vi "Actor Core.vi"(8 "error in":errorcluster, 11 "Pic Json Generator in":refnum<class "Pic Json Generator.lvclass">) -> (0 "error out":errorcluster, 3 "Actor out":refnum<class "Actor.lvclass">)   [LabVIEW 2018, in "Pic Json Generator.lvlib" / "Pic Json Generator.lvclass"]
doc: "The user interface for this panel.\n\n----\nPlease see the following web address for additional documentation and tutorial information:\nhttp://www.mooregoodideas.com/mgi-panel-manager/\n\nAuthor: Derek Trepanier\n\nCopyright (c) 2018, Moore Good Ideas, Inc.\n\nAll rights reserved.\n\nRedistribution and use in source and binary forms, with or without modification, are permitted provided that the following conditions are met:\n\n * Redistributions of source code must retain the above copyright notice, this list of conditions and the following disclaimer.\n * Redistributions in binary form must reproduce the above copyright notice, this list of conditions and the following disclaimer in the documentation and/or other materials provided with the distribution.\n * Neither the name of Moore Good Ideas, Inc. nor the names of its contributors may be used to endorse or promote products derived from this software without specific prior written permission.\n\nTHIS SOFTWARE IS PROVIDED BY THE COPYRIGHT HOLDERS AND CONTRIBUTORS \"AS IS\" AND ANY EXPRESS OR IMPLIED WARRANTIES, INCLUDING, BUT NOT LIMITED TO, THE IMPLIED WARRANTIES OF MERCHANTABILITY AND FITNESS FOR A PARTICULAR PURPOSE ARE DISCLAIMED. IN NO EVENT SHALL THE COPYRIGHT OWNER OR CONTRIBUTORS BE LIABLE FOR ANY DIRECT, INDIRECT, INCIDENTAL, SPECIAL, EXEMPLARY, OR CONSEQUENTIAL DAMAGES (INCLUDING, BUT NOT LIMITED TO, PROCUREMENT OF SUBSTITUTE GOODS OR SERVICES; LOSS OF USE, DATA, OR PROFITS; OR BUSINESS INTERRUPTION) HOWEVER CAUSED AND ON ANY THEORY OF LIABILITY, WHETHER IN CONTRACT, STRICT LIABILITY, OR TORT (INCLUDING NEGLIGENCE OR OTHERWISE) ARISING IN ANY WAY OUT OF THE USE OF THIS SOFTWARE, EVEN IF ADVISED OF THE POSSIBILITY OF SUCH DAMAGE."
uses:
  Pic Json Generator.lvclass
  C:/Program Files (x86)/National Instruments/LabVIEW 2018/vi.lib/MGI/Panel Manager/Panel Actor/Panel Actor/Panel Actor.lvclass
  C:/Program Files (x86)/National Instruments/LabVIEW 2018/vi.lib/ActorFramework/Actor/Actor.lvclass
  <vilib>/ActorFramework/Actor/Actor.lvclass
  Pic Json Generator.lvclass/Pic Json Generator.ctl
  <vilib>/ActorFramework/Actor/Actor.lvclass/Actor.ctl
  <vilib>/ActorFramework/Message Enqueuer/Message Enqueuer.lvclass/Message Enqueuer.ctl
  <vilib>/ActorFramework/Message Enqueuer/Init from Existing Queue.vi
  <vilib>/ActorFramework/Message Enqueuer/Enqueue.vi
  <vilib>/ActorFramework/Stop Msg/Stop Msg.lvclass
  C:/Program Files (x86)/National Instruments/LabVIEW 2018/vi.lib/ActorFramework/Message/Message.lvclass
  <vilib>/ActorFramework/Message Priority Queue/Priority Enqueue.vi
  <vilib>/ActorFramework/Message Enqueuer/Message Enqueuer.lvclass
  <vilib>/MGI/Panel Manager/Panel Actor/Panel Actor/Panel Actor.lvclass
panel:
  out "Frame Height":u32
  out "Frame Width":u32
  out "End Frame Num":u32
  in  "Generate":bool
  in  "Start Frame Num":u32
  in  "Num of Row":u32
  in  "Num of Column":u32
  in  "Pic File Path":path
  in  "Data File Path":path
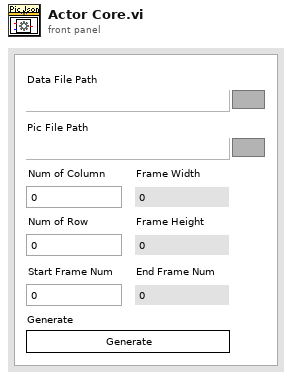
[diagram p1: front panel]
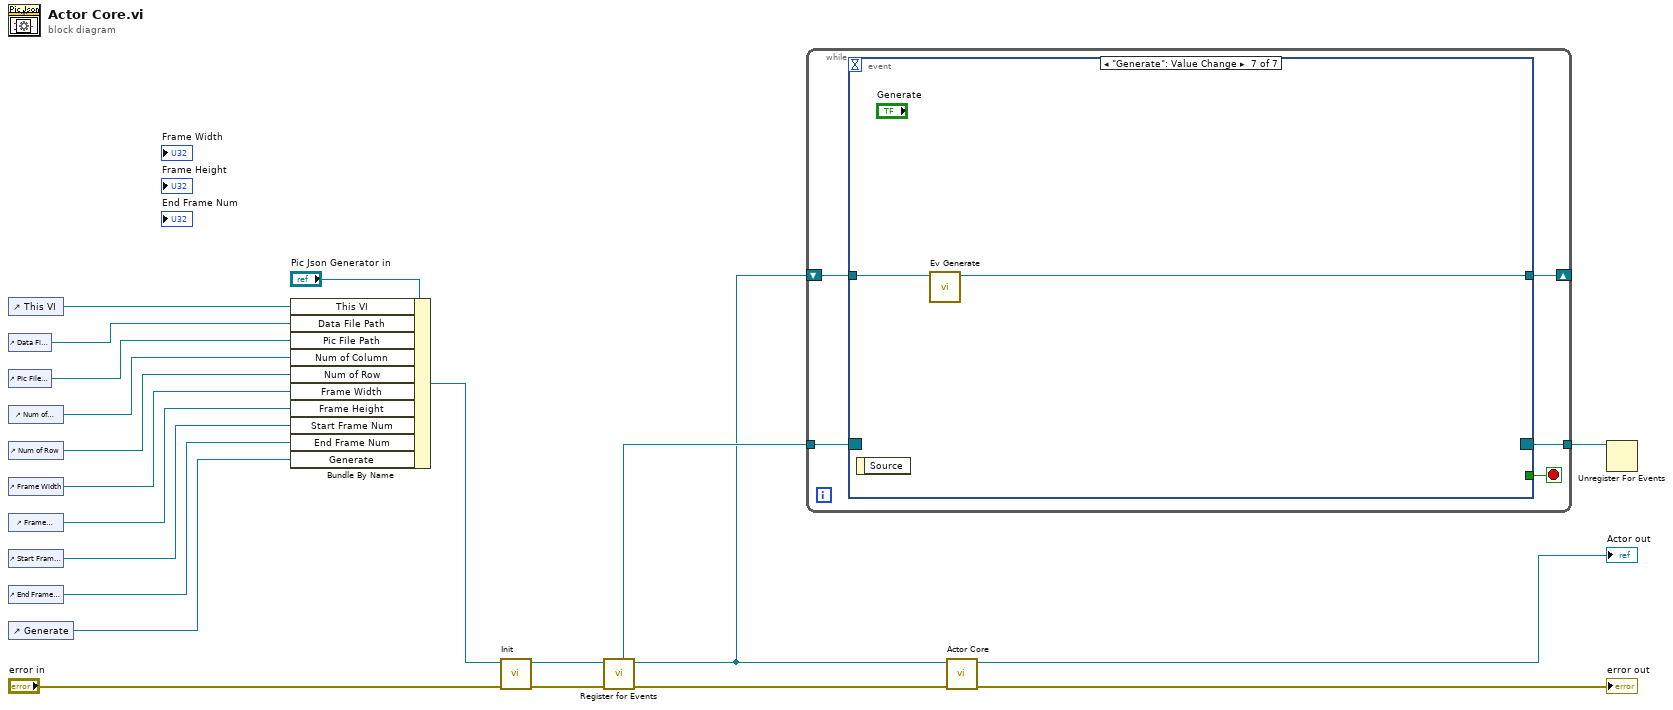
[diagram p0: block diagram]
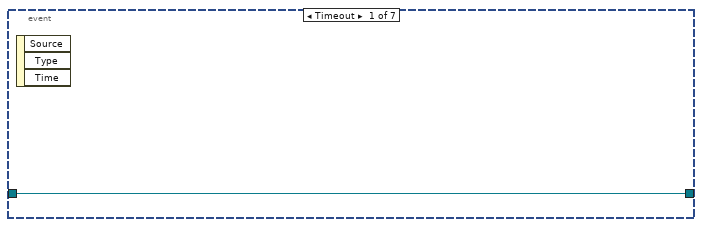
[diagram p2: hidden frame]
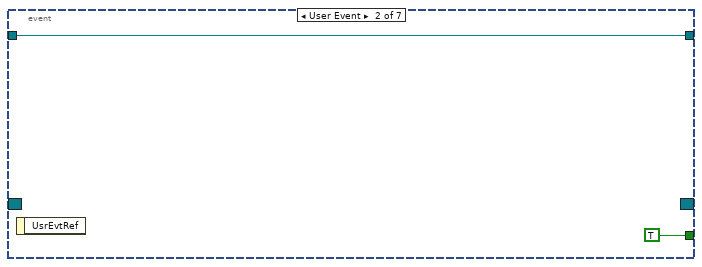
[diagram p3: hidden frame]
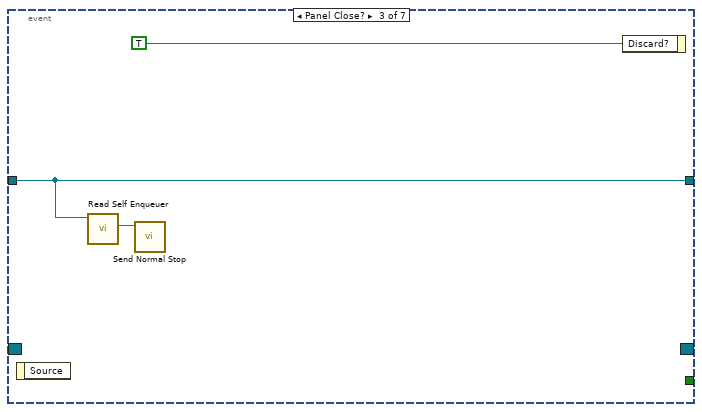
[diagram p4: hidden frame]
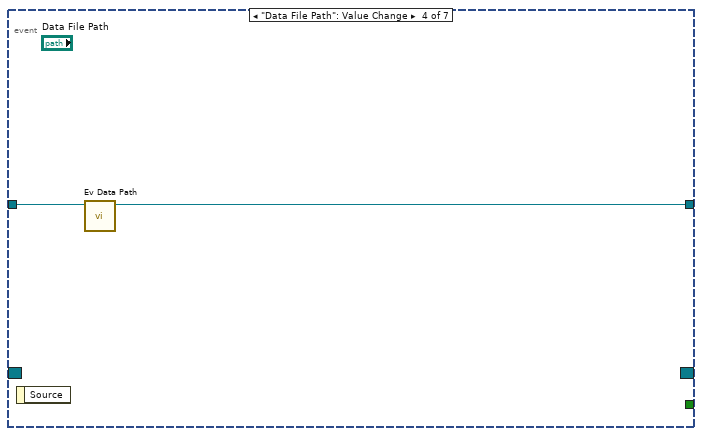
[diagram p5: hidden frame]
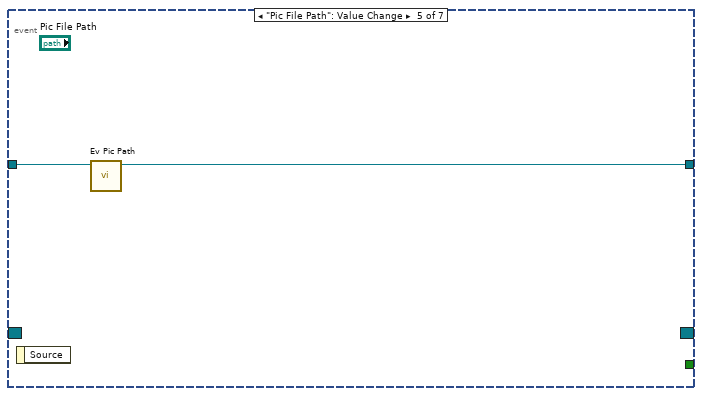
[diagram p6: hidden frame]
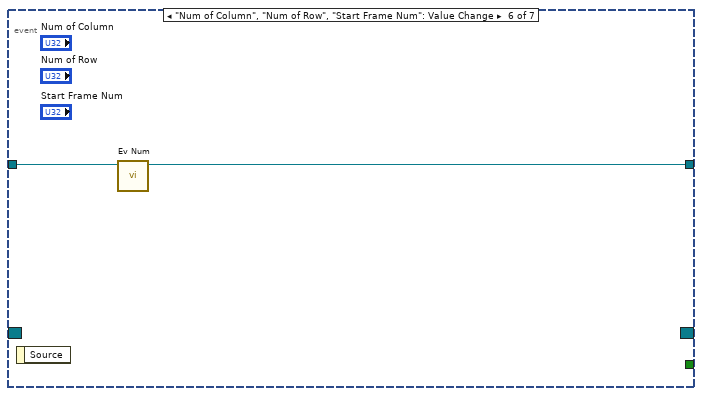
[diagram p7: hidden frame]
diagram:
  n1 = control-ref of="This VI"() -> (w1:refnum<vi>)
  n2 = control-ref of="Data File Path"() -> (w11:refnum<vi>)
  n3 = control-ref of="Pic File Path"() -> (w10:refnum<vi>)
  n4 = control-ref of="Num of Column"() -> (w7:refnum<vi>)
  n5 = control-ref of="Num of Row"() -> (w6:refnum<vi>)
  n6 = control-ref of="Frame Width"() -> (w5:refnum<vi>)
  n7 = control-ref of="Frame Height"() -> (w4:refnum<vi>)
  n8 = control-ref of="Start Frame Num"() -> (w3:refnum<vi>)
  n9 = control-ref of="End Frame Num"() -> (w2:refnum<vi>)
  n10 = control-ref of="Generate"() -> (w9:refnum<vi>)
  n11 = Bundle By Name(cluster="Pic Json Generator in", "This VI"=w1, "Data File Path"=w11, "Pic File Path"=w10, "Num of Column"=w7, "Num of Row"=w6, "Frame Width"=w5, "Frame Height"=w4, "Start Frame Num"=w3, "End Frame Num"=w2, "Generate"=w9) -> (w8:refnum<class "Pic Json Generator.lvclass">)
  n12 = call "Init.vi"("error in (no error)"="error in", "Pic Json Generator in"=w8) -> ("error out"=w17:errorcluster, "Pic Json Generator out"=w18:refnum<class "Pic Json Generator.lvclass">)  [unwired: 8 in]
  n13 = call <vilib>:"Register for Events.vi"("Error In"=w17, "Panel Actor in"=w18) -> ("Error Out"=w16:errorcluster, "Panel Actor out"=w13:refnum<class "Pic Json Generator.lvclass">, "Pnl Actor"=w14:refnum<event-registration>)  [unwired: 6 in, 1 out]
  n14 = while {
    tunnel: w14 -> [w26]
    tunnel: [w24] -> w15
    shift-right: [w22] -> _
    shift-left: w13 -> [w23]
    stop <- w25 stop-if-true
    n15 = event shown="[6] \"Generate\": Value Change" {
      selector: w26 -> [_ _ _ _ _ _ _]
      dyn-events: [_ _ _ _ _ _ _] -> w24
      timeout: _ -> [_ _ _ _ _ _ _]
      tunnel: [_ TRUE _ _ _ _ _] -> w25
      tunnel: w23 -> [w27 w28 w30 w34 w36 w38 w40]
      tunnel: [w27 w28 w30 w33 w35 w37 w39] -> w22
      event Timeout {
        n16 = event-data() -> ()  [unwired: 1 in, 3 out]
      }
      event User Event {
        n17 = event-data() -> ()  [unwired: 1 in, 1 out]
      }
      event Panel Close? {
        n18 = event-data() -> ()  [unwired: 1 in, 1 out]
        n19 = call <vilib>:"Read Self Enqueuer.vi"("Actor"=w30) -> ("Self Enqueuer"=w31:refnum<class "Message Enqueuer.lvclass">)  [unwired: 10 in]
        n20 = call <vilib>:"Send Normal Stop.vi"("Message Enqueuer"=w31) -> ()  [unwired: 10 in, 1 out]
        n21 = event-data("Discard?"=TRUE) -> ()  [unwired: 1 in, 1 out]
      }
      event "Data File Path": Value Change {
        n22 = event-data() -> ()  [unwired: 1 in, 1 out]
        n23 = call "Ev Data Path.vi"("Pic Json Generator in"=w34) -> ("Pic Json Generator out"=w33:refnum<class "Pic Json Generator.lvclass">)  [unwired: 9 in, 1 out]
      }
      event "Pic File Path": Value Change {
        n24 = event-data() -> ()  [unwired: 1 in, 1 out]
        n25 = call "Ev Pic Path.vi"("Pic Json Generator in"=w36) -> ("Pic Json Generator out"=w35:refnum<class "Pic Json Generator.lvclass">)  [unwired: 9 in, 1 out]
      }
      event "Num of Column", "Num of Row", "Start Frame Num": Value Change {
        n26 = event-data() -> ()  [unwired: 1 in, 1 out]
        n27 = call "Ev Num.vi"("Pic Json Generator in"=w38) -> ("Pic Json Generator out"=w37:refnum<class "Pic Json Generator.lvclass">)  [unwired: 9 in, 1 out]
      }
      event "Generate": Value Change {
        n28 = event-data() -> ()  [unwired: 1 in, 1 out]
        n29 = call "Ev Generate.vi"("Pic Json Generator in"=w40) -> ("Pic Json Generator out"=w39:refnum<class "Pic Json Generator.lvclass">)  [unwired: 9 in, 1 out]
      }
    }
  }
  n30 = call-parent "Actor Core.vi"("error in"=w16, "Panel Actor in"=w13) -> ("error out"=→"error out":errorcluster, "Actor out"=→"Actor out":refnum<class "Actor.lvclass">)  [unwired: 8 in]
  n31 = Unregister For Events(event registration refnum=w15) -> ()  [unwired: 1 in, 1 out]
